vi "UTILITY VI Path Tester.vi"() -> ()   [LabVIEW 2014]
uses:
  <vilib>/Platform/fileVersionInfo.llb/FileVersionInformation.ctl
panel:
  out "FileVersionInfo Out":T1
  out "File Version Info":string
  out "current path":path
  out "Application:Kind":T2(ring)
  out "Robocopy Path":string
  out "Folder Path":path
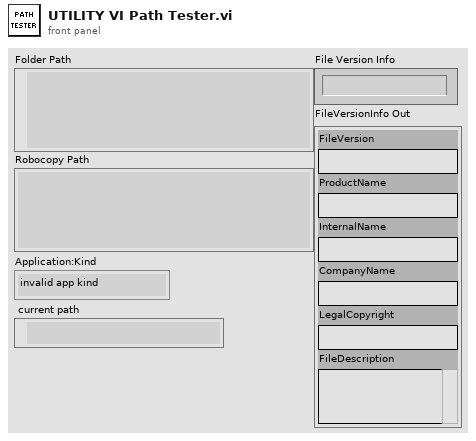
[diagram p1: front panel]
types:
  T1 = typedef "FileVersionInformation.ctl" = cluster{"FileVersion":string, "ProductName":string, "InternalName":string, "CompanyName":string, "LegalCopyright":string, "FileDescription":string}
  T2 = enum32{"invalid app kind", "Development System", "Run Time System", "Student Edition", "Embedded LabVIEW", "Evaluation", "Custom"}
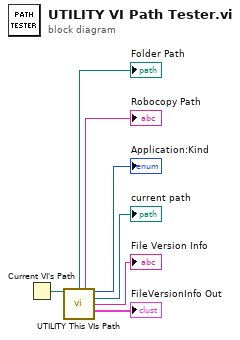
[diagram p0: block diagram]
diagram:
  n1 = Current VI's Path() -> (path=w7:path)
  n2 = call "UTILITY This VIs Path.vi"("path"=w7) -> ("Folder Path"=→"Folder Path":path, "Robocopy Path"=→"Robocopy Path":string, "Application:Kind"=→"Application:Kind":T2, "current path"=→"current path":path, "File Version Info"=→"File Version Info":string, "FileVersionInfo Out"=→"FileVersionInfo Out":T1)  [unwired: 8 in, 1 out]
